vi "PH_Timing.set Head Attributes.vi"(1 "GUI Refs Heads":T1) -> (0 "Heads":T2[](array[typedef]) {"GD"."Device Status" items=["no info", "off/false/out", "on/true/in", "Failure", "Alarm", "Status 1", "Status 2", "Status 3"]; "Data"."CH" items=["System (To)", "Channel A", "Channel B", "Channel C", "Channel D", "Channel E", "Channel F", "Channel G", "Channel H"]; "Data"."Delay" format="%#_7f"})   [LabVIEW 2014, in "PH_Timing.lvlib"]
doc: "In this VI the related instances which are not set in the Read DB Vi are defined and set (includinbg default values) to own attributes."
uses:
  PH_Timing.lvlib
  PH_Timing.PU Data.ctl
  PH_Timing.PU Info.ctl
  PH_Basics/PH_StatusHandler/PH_StatusHandler.Status.ctl
  PH_Basics/PH_PP_Common/PH_PP_Common.PUs.ctl
  PH_Basics/PH_StatusHandler/PH_StatusHandler.lvlib
  PH_Basics/PH_PP_Common/PH_PP_Common.lvlib
panel:
  # "s"
  # "s"
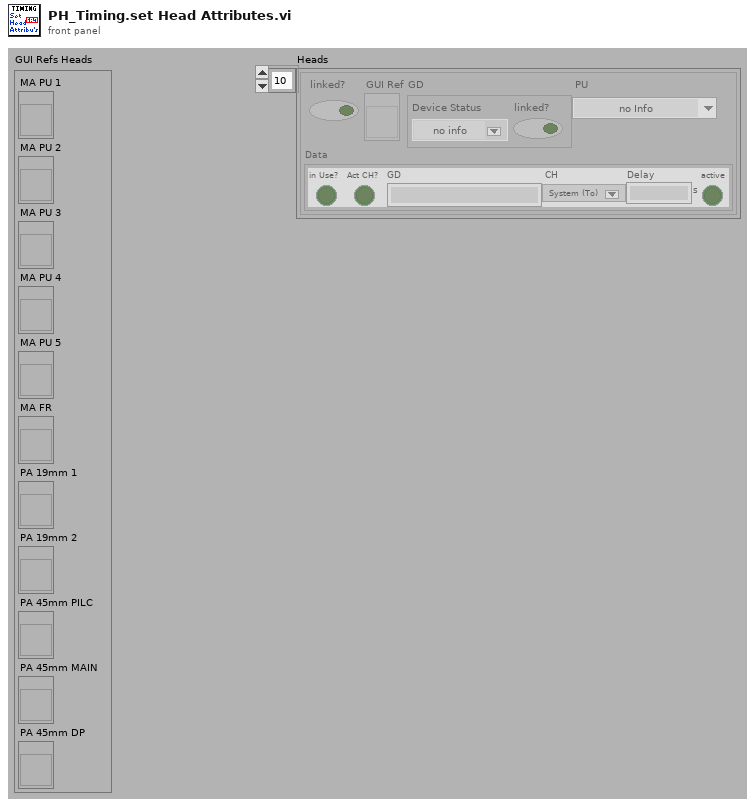
[diagram p1: front panel]
types:
  T1 = cluster{"MA PU 1":refnum<vi>, "MA PU 2":refnum<vi>, "MA PU 3":refnum<vi>, "MA PU 4":refnum<vi>, "MA PU 5":refnum<vi>, "MA FR":refnum<vi>, "PA 19mm 1":refnum<vi>, "PA 19mm 2":refnum<vi>, "PA 45mm PILC":refnum<vi>, "PA 45mm MAIN":refnum<vi>, "PA 45mm DP":refnum<vi>}
  T2 = typedef "PH_Timing.lvlib/PH_Timing.PU Data.ctl" = cluster{"linked?":bool, "Data":T3, "GD":cluster{"Device Status":T4, "linked?":bool}, "GUI Ref":refnum<vi>, "PU":T5}
  T3 = typedef "PH_Timing.lvlib/PH_Timing.PU Info.ctl" = cluster{"Act CH?":bool, "GD":string, "CH":i32, "Delay":dbl, "active":bool, "in Use?":bool}
  T4 = typedef "PH_StatusHandler.lvlib/PH_StatusHandler.Status.ctl" = i16
  T5 = typedef "PH_PP_Common.lvlib/PH_PP_Common.PUs.ctl" = enum16{"no Info", "PA-19mm-1", "PA-19mm-2", "PA-45mm-PILC", "PA-45mm-MAIN", "MA-PU-1", "MA-PU-2", "MA-PU-3", "MA-PU-4", "MA-PU-5", "MA-PU-6", "MA-FR", "MA-PILC", "PA-45mm-DP"}
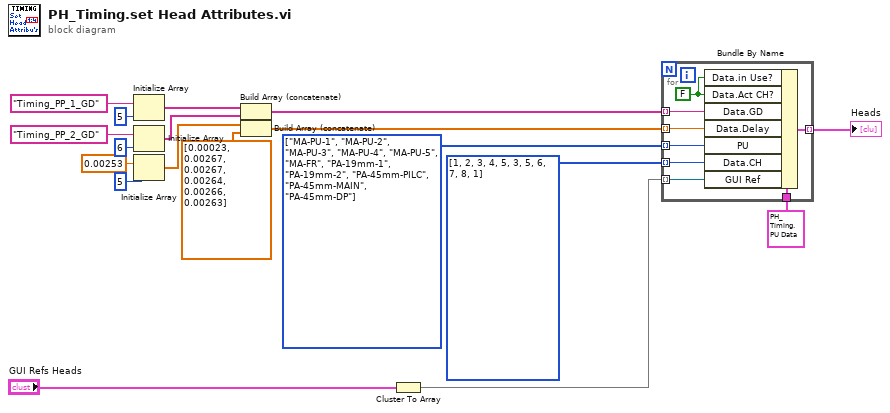
[diagram p0: block diagram]
diagram:
  w14 = T5[] [enum."MA-PU-1", enum."MA-PU-2", enum."MA-PU-3", enum."MA-PU-4", enum."MA-PU-5", enum."MA-FR", enum."PA-19mm-1", enum."PA-19mm-2", enum."PA-45mm-PILC", enum."PA-45mm-MAIN", enum."PA-45mm-DP"] items=["no Info", "PA-19mm-1", "PA-19mm-2", "PA-45mm-PILC", "PA-45mm-MAIN", "MA-PU-1", "MA-PU-2", "MA-PU-3", "MA-PU-4", "MA-PU-5", "MA-PU-6", "MA-FR", "MA-PILC", "PA-45mm-DP"]
  w18 = i32[] [1, 2, 3, 4, 5, 3, 5, 6, 7, 8, 1] items=["System (To)", "Channel A", "Channel B", "Channel C", "Channel D", "Channel E", "Channel F", "Channel G", "Channel H"]
  n1 = Initialize Array("Timing_PP_1_GD", 5) -> (w13:string[])
  n2 = Initialize Array("Timing_PP_2_GD", 6 ("dimension size")) -> (w12:string[])
  n3 = Initialize Array(0.00253 ("PU Delay"), 5 ("dimension size")) -> (w10:dbl[])
  n4 = Build Array (concatenate)(w13, w12) -> (w17:string[])
  n5 = Build Array (concatenate)(w10, dbl[] [0.00023, 0.00267, 0.00267, 0.00264, 0.00266, 0.00263]) -> (w15:dbl[])
  n6 = Cluster To Array(cluster="GUI Refs Heads") -> (array=w3:refnum<vi>[])
  n7 = for {
    tunnel: [w26] -> w5 mode=indexing
    tunnel: w18 -> [w21] mode=indexing
    tunnel: w17 -> [w25] mode=indexing
    tunnel: w15 -> [w24] mode=indexing
    tunnel: w14 -> [w20] mode=indexing
    tunnel: T2 {"linked?"=FALSE, "Data"={"Act CH?"=FALSE, "GD"="N/A", "CH"=1, "Delay"=99999.0, "active"=FALSE, "in Use?"=FALSE}, "GD"={"Device Status"=0, "linked?"=FALSE}, "GUI Ref"=refnum, "PU"=enum."no Info"} ("PU Data Info") -> [w23]
    tunnel: w3 -> [w19] mode=indexing
    w22 = FALSE ("Data.activate Channel?")
    n8 = Bundle By Name(cluster=w23, "Data.in Use?"=w22, "Data.Act CH?"=w22, "Data.GD"=w25, "Data.Delay"=w24, "PU"=w20, "Data.CH"=w21, "GUI Ref"=w19) -> (w26:T2)
  }
  "Heads" <- w5
